vi "Lab2 - Ines.vi"() -> ()   [LabVIEW 2025]
panel:
  in  "Angle (degrees)":dbl=1.0 min=1.0 max=89.0
  in  "Initial height (m)":dbl min=0.0
  in  "Initial speed (m/s) 2":dbl=1.0 min=1.0
  out "Y Position vs. X Position":cluster{"Y":dbl[], "Y":dbl[]}[](graph)
  out "Y Position vs. T":cluster{"Y":dbl[], "Y":dbl[]}[](graph)
  out "X Position vs. T":cluster{"Y":dbl[], "Y":dbl[]}[](graph)
  in  "ADD RUN":bool
  # "Ines Front Pannel"
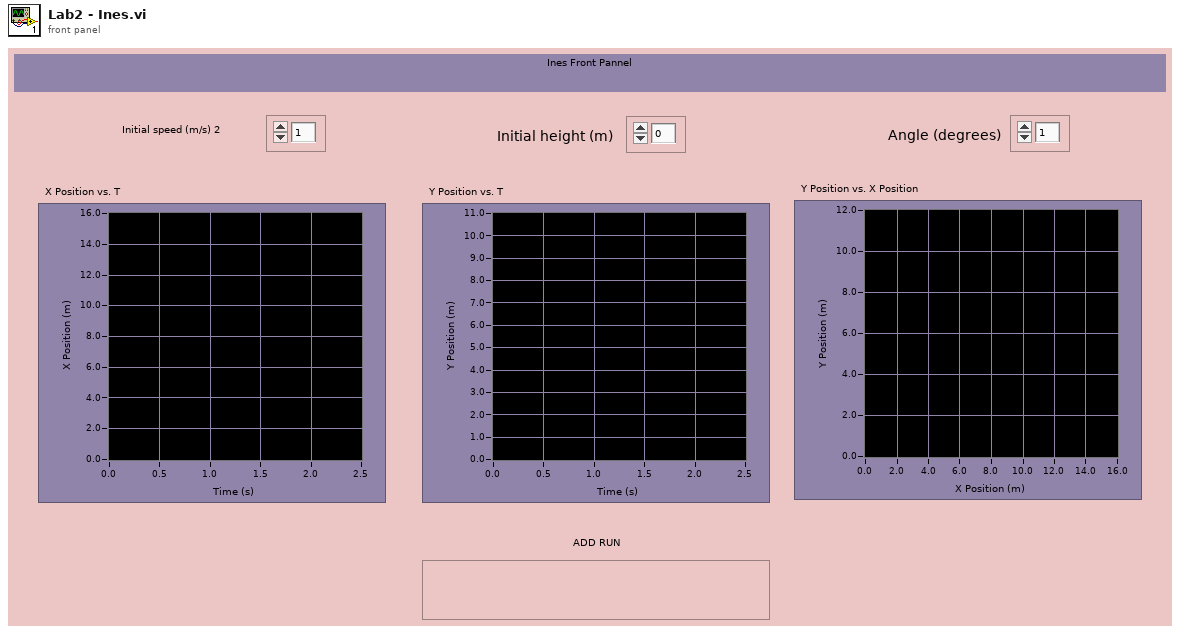
[diagram p1: front panel]
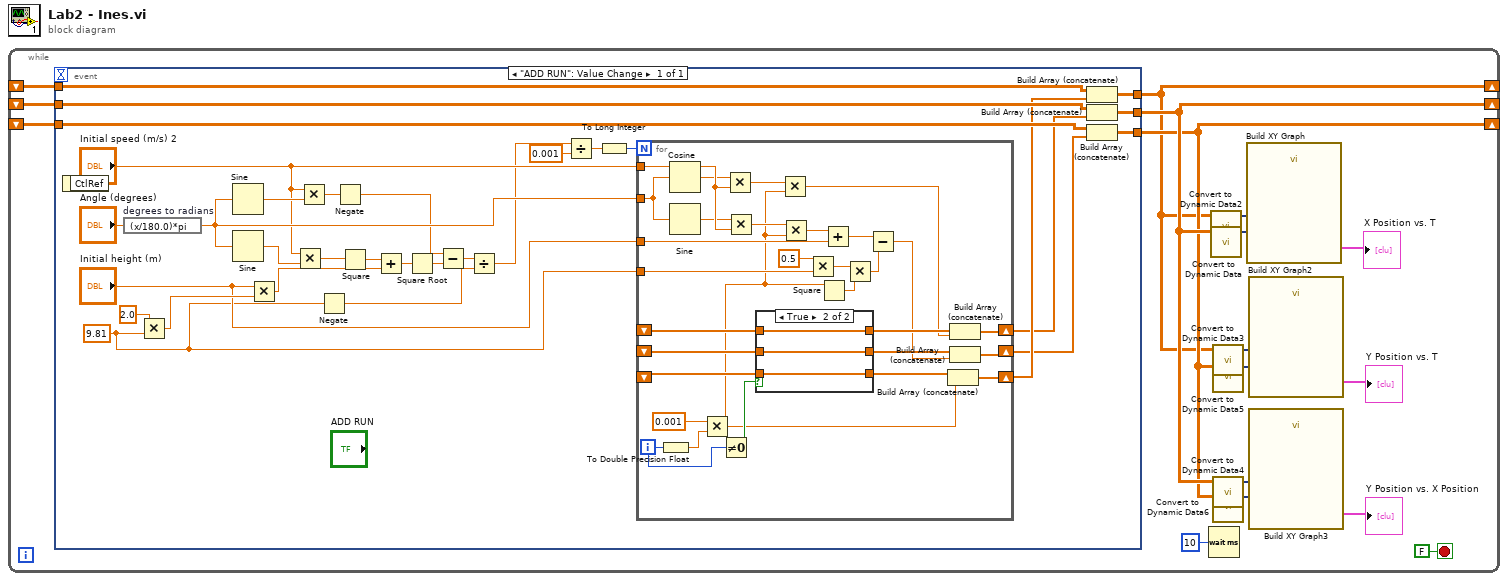
[diagram p0: block diagram]
diagram:
  n1 = while {
    shift-right: [w6] -> _
    shift-left: _ -> [w15]
    shift-right: [w3] -> _
    shift-left: _ -> [w14]
    shift-right: [w1] -> _
    shift-left: _ -> [w13]
    stop <- FALSE stop-if-true
    n2 = event shown="[0] \"ADD RUN\": Value Change" {
      selector: _ -> [_]
      dyn-events: _ -> [_]
      timeout: _ -> [_]
      tunnel: [w48] -> w6
      tunnel: w15 -> [w47]
      tunnel: [w46] -> w3
      tunnel: w14 -> [w45]
      tunnel: [w44] -> w1
      tunnel: w13 -> [w43]
      event "ADD RUN": Value Change {
        w18 = 9.81
        n3 = event-data() -> ()  [unwired: 1 in, 1 out]
        n4 = expression code="(x/180.0)*pi" "degrees to radians"("Angle (degrees)") -> (w33:dbl)
        n5 = Multiply(x=2.0, y=w18) -> (x*y=w29:dbl)
        n6 = Sine(x=w33) -> (sin(x)=w35:dbl)
        n7 = Sine(x=w33) -> (sin(x)=w31:dbl)
        n8 = Multiply(x="Initial height (m)", y=w29) -> (x*y=w26:dbl)
        n9 = Multiply(x="Initial speed (m/s) 2", y=w31) -> (x*y=w30:dbl)
        n10 = Multiply(x="Initial speed (m/s) 2", y=w35) -> (x*y=w34:dbl)
        n11 = Negate(x=w18) -> (-x=w21:dbl)
        n12 = Negate(x=w34) -> (-x=w24:dbl)
        n13 = Square(x=w30) -> (x^2=w27:dbl)
        n14 = Add(x=w27, y=w26) -> (x+y=w25:dbl)
        n15 = Square Root(x=w25) -> (sqrt(x)=w23:dbl)
        n16 = Subtract(x=w24, y=w23) -> (x-y=w22:dbl)
        n17 = Divide(x=w22, y=w21) -> (x/y=w20:dbl)
        n18 = Divide(x=w20, y=0.001) -> (x/y=w40:dbl)
        n19 = To Long Integer(number=w40) -> (32bit integer=w39:i32)
        n20 = for {
          N: w39 -> [_]
          tunnel: "Initial speed (m/s) 2" -> [w64]
          tunnel: "Initial height (m)" -> [w57]
          tunnel: w33 -> [w65]
          tunnel: w18 -> [w54]
          shift-right: [w76] -> w36
          shift-left: _ -> [w68]
          shift-right: [w75] -> w37
          shift-left: _ -> [w70]
          shift-right: [w74] -> w38
          shift-left: _ -> [w67]
          i -> [w72]
          n21 = To Double Precision Float(number=w72) -> (double precision float=w77:dbl)
          n22 = Cosine(x=w65) -> (cos(x)=w63:dbl)
          n23 = Sine(x=w65) -> (sin(x)=w62:dbl)
          n24 = Multiply(x=0.001, y=w77) -> (x*y=w50:dbl)
          n25 = Not Equal To 0?(x=w72) -> (x != 0?=w73:bool)
          n26 = Multiply(x=w63, y=w64) -> (x*y=w61:dbl)
          n27 = Multiply(x=w62, y=w64) -> (x*y=w59:dbl)
          n28 = case shown="True" w73 {
            tunnel: [_ w81] -> w71
            tunnel: w70 -> [_ w81]
            tunnel: [_ w80] -> w69
            tunnel: w68 -> [_ w80]
            tunnel: [_ w79] -> w66
            tunnel: w67 -> [_ w79]
            frame False {
            }
            frame True {
            }
          }
          n29 = Multiply(x=w61, y=w50) -> (x*y=w60:dbl)
          n30 = Multiply(x=w59, y=w50) -> (x*y=w58:dbl)
          n31 = Multiply(x=0.5, y=w54) -> (x*y=w52:dbl)
          n32 = Square(x=w50) -> (x^2=w51:dbl)
          n33 = Add(x=w58, y=w57) -> (x+y=w56:dbl)
          n34 = Multiply(x=w52, y=w51) -> (x*y=w49:dbl)
          n35 = Subtract(x=w56, y=w49) -> (x-y=w55:dbl)
          n36 = Build Array (concatenate)(w66, w50) -> (w74:dbl[])
          n37 = Build Array (concatenate)(w71, w60) -> (w75:dbl[])
          n38 = Build Array (concatenate)(w69, w55) -> (w76:dbl[])
        }
        n39 = Build Array (concatenate)(w43, w38) -> (w44:dbl[][])
        n40 = Build Array (concatenate)(w47, w37) -> (w48:dbl[][])
        n41 = Build Array (concatenate)(w45, w36) -> (w46:dbl[][])
      }
    }
    n42 = Wait (ms)(milliseconds to wait=u32 10) -> ()  [unwired: 1 out]
    n43 = call "Convert to Dynamic Data2"("2D Array"=w1) -> ("Dynamic Data Type"=w10:dynamicdata)  [unwired: 3 in]
    n44 = call "Convert to Dynamic Data"("2D Array"=w6) -> ("Dynamic Data Type"=w11:dynamicdata)  [unwired: 3 in]
    n45 = call "Convert to Dynamic Data3"("2D Array"=w1) -> ("Dynamic Data Type"=w7:dynamicdata)  [unwired: 3 in]
    n46 = call "Convert to Dynamic Data5"("2D Array"=w3) -> ("Dynamic Data Type"=w4:dynamicdata)  [unwired: 3 in]
    n47 = call "Convert to Dynamic Data4"("2D Array"=w6) -> ("Dynamic Data Type"=w5:dynamicdata)  [unwired: 3 in]
    n48 = call "Convert to Dynamic Data6"("2D Array"=w3) -> ("Dynamic Data Type"=w2:dynamicdata)  [unwired: 3 in]
    n49 = call "Build XY Graph"("Y Input"=w11, "X Input"=w10) -> ("XY Graph"=→"X Position vs. T":cluster{"X":dbl[], "Y":dbl[]}[])  [unwired: 8 in, 1 out]
    n50 = call "Build XY Graph2"("Y Input"=w4, "X Input"=w7) -> ("XY Graph"=→"Y Position vs. T":cluster{"X":dbl[], "Y":dbl[]}[])  [unwired: 8 in, 1 out]
    n51 = call "Build XY Graph3"("Y Input"=w2, "X Input"=w5) -> ("XY Graph"=→"Y Position vs. X Position":cluster{"X":dbl[], "Y":dbl[]}[])  [unwired: 8 in, 1 out]
  }
